vi "4.7.vi"() -> ()   [LabVIEW 2017]
panel:
  out "数值 2":dbl
  out "循环次数":i32
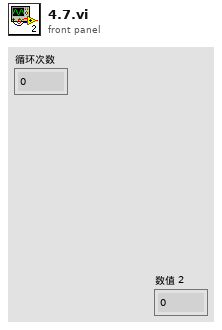
[diagram p1: front panel]
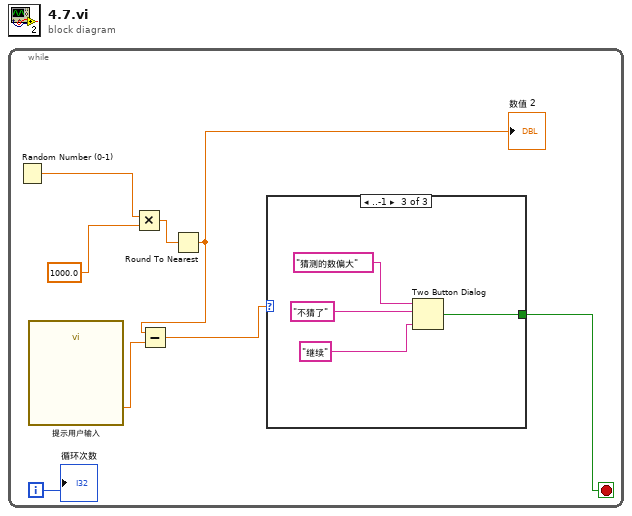
[diagram p0: block diagram]
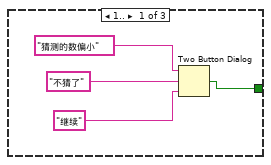
[diagram p2: hidden frame]
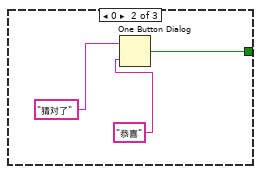
[diagram p3: hidden frame]
diagram:
  n1 = while {
    i -> [w5]
    stop <- w3 stop-if-true
    n2 = Random Number (0-1)() -> (number: 0 to 1=w8:dbl)
    n3 = call "提示用户输入"() -> ("请在1-1000内猜"=w2:dbl)  [unwired: 17 in, 2 out]
    n4 = Multiply(x=w8, y=1000.0 ("数字(0-1)")) -> (x*y=w6:dbl)
    n5 = Round To Nearest(number=w6) -> (nearest integer value=w4:dbl)
    "数值 2" <- w4
    n6 = Subtract(x=w4, y=w2) -> (x-y=w1:dbl)
    n7 = case shown="..-1" w1 {
      tunnel: [w11 w14 w18] -> w3
      frame 1.. {
        n8 = Two Button Dialog(message="猜测的数偏小", 1:"继续", 2:"不猜了") -> (T button?=w11:bool)
      }
      frame 0 {
        n9 = One Button Dialog(message="猜对了", button name ("OK")="恭喜") -> (true=w14:bool)
      }
      frame ..-1 {
        n10 = Two Button Dialog(message="猜测的数偏大", 1:"继续", 2:"不猜了") -> (T button?=w18:bool)
      }
    }
    "循环次数" <- w5
  }
